vi "Phase_Shift_Keying.vi"() -> ()   [LabVIEW 2019]
panel:
  out "Modulated Signal":dbl[](graph)=[0.0, 0.40673664307580015, 0.7431448254773941, 0.9510565162951535, 0.9945218953682734, 0.8660254037844386, 0.5877852522924732, 0.20791169081775887, -0.20791169081775907, -0.5877852522924734, -0.8660254037844388, -0.9945218953682734, -0.9510565162951536, -0.7431448254773946, -0.4067366430757993, -2.4492935982947064e-16, 0.4067366430757997, 0.7431448254773948, 0.9510565162951538, 0.9945218953682733, 0.8660254037844383, 0.5877852522924734, 0.20791169081775912, -0.2079116908177584, -0.5877852522924728, -0.8660254037844387, -0.9945218953682732, -0.9510565162951538, -0.743144825477393, -0.40673664307579954, -4.898587196589413e-16, 0.40673664307580026, 0.7431448254773935, 0.9510565162951534, 0.9945218953682732, 0.8660254037844384, 0.5877852522924721, 0.20791169081775934, -0.2079116908177599, -0.5877852522924726, -0.8660254037844395, -0.9945218953682734, -0.9510565162951538, -0.7431448254773931, -0.40673664307579976, -7.347880794884119e-16, 0.40673664307579843, 0.7431448254773945, 0.9510565162951533, 0.9945218953682735, 0.8660254037844385, 0.5877852522924709, 0.2079116908177613, -0.20791169081775965, -0.5877852522924725, -0.8660254037844394, -0.9945218953682737, -0.9510565162951539, -0.7431448254773934, -0.4067366430758, -9.797174393178826e-16, 0.4067366430757982, 0.7431448254773944, 0.9510565162951543, 0.9945218953682736, 0.8660254037844386, 0.587785252292474, 0.2079116908177581, -0.2079116908177629, -0.5877852522924722, -0.8660254037844393, -0.9945218953682733, -0.9510565162951529, -0.7431448254773958, -0.4067366430758002, 2.328066879653148e-15, -0.40673664307580126, -0.7431448254773966, -0.9510565162951532, -0.9945218953682732, -0.8660254037844369, -0.5877852522924742, -0.20791169081775834, 0.2079116908177557, 0.587785252292472, 0.8660254037844392, 0.9945218953682737, 0.951056516295154, 0.7431448254773936, 0.4067366430757972, 1.4695761589768238e-15, -0.40673664307580104, -0.7431448254773916, -0.9510565162951531, -0.9945218953682733, -0.866025403784437, -0.5877852522924744, -0.20791169081775857, 0.20791169081775546, 0.5877852522924776, 0.866025403784439, 0.994521895368273, 0.9510565162951519, 0.7431448254773938, 0.4067366430758039, -5.3909218387947074e-15, -0.4067366430758008, -0.7431448254773915, -0.951056516295153, -0.9945218953682733, -0.8660254037844372, -0.5877852522924746, -0.20791169081775185, 0.20791169081776217, 0.5877852522924716, 0.8660254037844354, 0.9945218953682736, 0.9510565162951542, 0.7431448254773939, 0.40673664307579765, 1.959434878635765e-15, -0.40673664307580054, -0.7431448254773912, -0.9510565162951552, -0.9945218953682733, -0.8660254037844408, -0.587785252292469, -0.20791169081775904, 0.20791169081775498, 0.5877852522924714, 0.8660254037844388, 0.9945218953682736, 0.9510565162951542, 0.7431448254773941, 0.4067366430757979, 2.204364238465236e-15, -0.4067366430758068, -0.7431448254773959, -0.9510565162951529, -0.9945218953682733, -0.8660254037844374, -0.587785252292475, -0.2079116908177593, 0.20791169081776167, 0.587785252292477, 0.8660254037844386, 0.9945218953682728, 0.9510565162951521, 0.7431448254773942, 0.4067366430758046, -4.656133759306296e-15, 0.4067366430758001, 0.7431448254773958, 0.9510565162951506, 0.9945218953682726, 0.866025403784441, 0.5877852522924751, 0.20791169081775954, -0.20791169081776145, -0.5877852522924768, -0.866025403784442, -0.9945218953682743, -0.9510565162951544, -0.7431448254773945, -0.4067366430757983, 4.411204399476825e-15, 0.4067366430757934, 0.7431448254774004, 0.9510565162951528, 0.9945218953682734, 0.8660254037844377, 0.5877852522924696, 0.20791169081775282, -0.20791169081775426, -0.5877852522924708, -0.8660254037844384, -0.9945218953682735, -0.9510565162951566, -0.7431448254773898, -0.40673664307580504, -2.9391523179536475e-15, 0.40673664307579965, 0.7431448254773955, 0.9510565162951549, 0.9945218953682742, 0.8660254037844343, 0.5877852522924756, 0.20791169081776, -0.20791169081776098, -0.5877852522924764, -0.8660254037844418, -0.9945218953682727, -0.9510565162951545, -0.7431448254773853, -0.40673664307579876, 3.921345679817883e-15, 0.40673664307579294, 0.7431448254773905, 0.951056516295157, 0.9945218953682734, 0.8660254037844379, 0.58778525229247, 0.2079116908177672, -0.2079116908177538, -0.5877852522924819, -0.8660254037844382, -0.9945218953682735, -0.9510565162951524, -0.7431448254773997, -0.4067366430757925, 1.0781843677589415e-14, 0.4067366430757992, 0.7431448254773951, 0.9510565162951503, 0.9945218953682742, 0.8660254037844345, 0.587785252292476, 0.20791169081776048, -0.20791169081776048, -0.5877852522924645, -0.8660254037844416, -0.9945218953682742, -0.9510565162951546, -0.743144825477395, -0.4067366430757862, 3.4314869601589423e-15, -0.4067366430758055, -0.7431448254773901, -0.9510565162951524, -0.9945218953682735, -0.8660254037844453, -0.5877852522924705, -0.20791169081775376, 0.2079116908177533, 0.58778525229247, 0.866025403784445, 0.9945218953682734, 0.9510565162951525, 0.7431448254773905, 0.4067366430758059, 3.91886975727153e-15, -0.40673664307581175, -0.7431448254773948, -0.9510565162951545, -0.9945218953682743, -0.8660254037844418, -0.5877852522924649, -0.20791169081776095, 0.20791169081776, 0.5877852522924756, 0.8660254037844343, 0.9945218953682742, 0.9510565162951504, 0.7431448254773955, 0.40673664307579965, -2.941628240500001e-15, -0.40673664307579205, -0.7431448254773994, -0.9510565162951523, -0.9945218953682735, -0.8660254037844384, -0.5877852522924824, -0.20791169081775426, 0.20791169081776673, 0.5877852522924696, 0.8660254037844377, 0.9945218953682734, 0.9510565162951571, 0.7431448254773908, 0.4067366430757934, 4.408728476930472e-15, -0.4067366430757983, -0.743144825477404, -0.9510565162951544, -0.9945218953682728, -0.866025403784442, -0.5877852522924768, -0.20791169081774755, 0.20791169081775954, 0.5877852522924751, 0.866025403784441, 0.9945218953682726, 0.951056516295155, 0.7431448254773863, 0.4067366430758001, -2.45176952084106e-15, -0.4067366430758046, -0.7431448254773895, -0.9510565162951565, -0.9945218953682721, -0.8660254037844386, -0.5877852522924712, -0.20791169081776864, 0.20791169081775235, 0.5877852522924807, 0.8660254037844374, 0.9945218953682733, 0.9510565162951529, 0.7431448254774007, 0.4067366430757938]
  out "Carrier Signal":dbl[](graph)=[0.0, 0.40673664307580015, 0.7431448254773941, 0.9510565162951535, 0.9945218953682734, 0.8660254037844386, 0.5877852522924732, 0.20791169081775887, -0.20791169081775907, -0.5877852522924734, -0.8660254037844388, -0.9945218953682734, -0.9510565162951536, -0.7431448254773946, -0.4067366430757993, -2.4492935982947064e-16, 0.4067366430757997, 0.7431448254773948, 0.9510565162951538, 0.9945218953682733, 0.8660254037844383, 0.5877852522924734, 0.20791169081775912, -0.2079116908177584, -0.5877852522924728, -0.8660254037844387, -0.9945218953682732, -0.9510565162951538, -0.743144825477393, -0.40673664307579954, -4.898587196589413e-16, 0.40673664307580026, 0.7431448254773935, 0.9510565162951534, 0.9945218953682732, 0.8660254037844384, 0.5877852522924721, 0.20791169081775934, -0.2079116908177599, -0.5877852522924726, -0.8660254037844395, -0.9945218953682734, -0.9510565162951538, -0.7431448254773931, -0.40673664307579976, -7.347880794884119e-16, 0.40673664307579843, 0.7431448254773945, 0.9510565162951533, 0.9945218953682735, 0.8660254037844385, 0.5877852522924709, 0.2079116908177613, -0.20791169081775965, -0.5877852522924725, -0.8660254037844394, -0.9945218953682737, -0.9510565162951539, -0.7431448254773934, -0.4067366430758, -9.797174393178826e-16, 0.4067366430757982, 0.7431448254773944, 0.9510565162951543, 0.9945218953682736, 0.8660254037844386, 0.587785252292474, 0.2079116908177581, -0.2079116908177629, -0.5877852522924722, -0.8660254037844393, -0.9945218953682733, -0.9510565162951529, -0.7431448254773958, -0.4067366430758002, 2.328066879653148e-15, 0.40673664307580126, 0.7431448254773966, 0.9510565162951532, 0.9945218953682732, 0.8660254037844369, 0.5877852522924742, 0.20791169081775834, -0.2079116908177557, -0.587785252292472, -0.8660254037844392, -0.9945218953682737, -0.951056516295154, -0.7431448254773936, -0.4067366430757972, -1.4695761589768238e-15, 0.40673664307580104, 0.7431448254773916, 0.9510565162951531, 0.9945218953682733, 0.866025403784437, 0.5877852522924744, 0.20791169081775857, -0.20791169081775546, -0.5877852522924776, -0.866025403784439, -0.994521895368273, -0.9510565162951519, -0.7431448254773938, -0.4067366430758039, 5.3909218387947074e-15, 0.4067366430758008, 0.7431448254773915, 0.951056516295153, 0.9945218953682733, 0.8660254037844372, 0.5877852522924746, 0.20791169081775185, -0.20791169081776217, -0.5877852522924716, -0.8660254037844354, -0.9945218953682736, -0.9510565162951542, -0.7431448254773939, -0.40673664307579765, -1.959434878635765e-15, 0.40673664307580054, 0.7431448254773912, 0.9510565162951552, 0.9945218953682733, 0.8660254037844408, 0.587785252292469, 0.20791169081775904, -0.20791169081775498, -0.5877852522924714, -0.8660254037844388, -0.9945218953682736, -0.9510565162951542, -0.7431448254773941, -0.4067366430757979, -2.204364238465236e-15, 0.4067366430758068, 0.7431448254773959, 0.9510565162951529, 0.9945218953682733, 0.8660254037844374, 0.587785252292475, 0.2079116908177593, -0.20791169081776167, -0.587785252292477, -0.8660254037844386, -0.9945218953682728, -0.9510565162951521, -0.7431448254773942, -0.4067366430758046, 4.656133759306296e-15, 0.4067366430758001, 0.7431448254773958, 0.9510565162951506, 0.9945218953682726, 0.866025403784441, 0.5877852522924751, 0.20791169081775954, -0.20791169081776145, -0.5877852522924768, -0.866025403784442, -0.9945218953682743, -0.9510565162951544, -0.7431448254773945, -0.4067366430757983, 4.411204399476825e-15, 0.4067366430757934, 0.7431448254774004, 0.9510565162951528, 0.9945218953682734, 0.8660254037844377, 0.5877852522924696, 0.20791169081775282, -0.20791169081775426, -0.5877852522924708, -0.8660254037844384, -0.9945218953682735, -0.9510565162951566, -0.7431448254773898, -0.40673664307580504, -2.9391523179536475e-15, 0.40673664307579965, 0.7431448254773955, 0.9510565162951549, 0.9945218953682742, 0.8660254037844343, 0.5877852522924756, 0.20791169081776, -0.20791169081776098, -0.5877852522924764, -0.8660254037844418, -0.9945218953682727, -0.9510565162951545, -0.7431448254773853, -0.40673664307579876, 3.921345679817883e-15, 0.40673664307579294, 0.7431448254773905, 0.951056516295157, 0.9945218953682734, 0.8660254037844379, 0.58778525229247, 0.2079116908177672, -0.2079116908177538, -0.5877852522924819, -0.8660254037844382, -0.9945218953682735, -0.9510565162951524, -0.7431448254773997, -0.4067366430757925, 1.0781843677589415e-14, 0.4067366430757992, 0.7431448254773951, 0.9510565162951503, 0.9945218953682742, 0.8660254037844345, 0.587785252292476, 0.20791169081776048, -0.20791169081776048, -0.5877852522924645, -0.8660254037844416, -0.9945218953682742, -0.9510565162951546, -0.743144825477395, -0.4067366430757862, 3.4314869601589423e-15, 0.4067366430758055, 0.7431448254773901, 0.9510565162951524, 0.9945218953682735, 0.8660254037844453, 0.5877852522924705, 0.20791169081775376, -0.2079116908177533, -0.58778525229247, -0.866025403784445, -0.9945218953682734, -0.9510565162951525, -0.7431448254773905, -0.4067366430758059, -3.91886975727153e-15, 0.40673664307581175, 0.7431448254773948, 0.9510565162951545, 0.9945218953682743, 0.8660254037844418, 0.5877852522924649, 0.20791169081776095, -0.20791169081776, -0.5877852522924756, -0.8660254037844343, -0.9945218953682742, -0.9510565162951504, -0.7431448254773955, -0.40673664307579965, 2.941628240500001e-15, 0.40673664307579205, 0.7431448254773994, 0.9510565162951523, 0.9945218953682735, 0.8660254037844384, 0.5877852522924824, 0.20791169081775426, -0.20791169081776673, -0.5877852522924696, -0.8660254037844377, -0.9945218953682734, -0.9510565162951571, -0.7431448254773908, -0.4067366430757934, -4.408728476930472e-15, 0.4067366430757983, 0.743144825477404, 0.9510565162951544, 0.9945218953682728, 0.866025403784442, 0.5877852522924768, 0.20791169081774755, -0.20791169081775954, -0.5877852522924751, -0.866025403784441, -0.9945218953682726, -0.951056516295155, -0.7431448254773863, -0.4067366430758001, 2.45176952084106e-15, 0.4067366430758046, 0.7431448254773895, 0.9510565162951565, 0.9945218953682721, 0.8660254037844386, 0.5877852522924712, 0.20791169081776864, -0.20791169081775235, -0.5877852522924807, -0.8660254037844374, -0.9945218953682733, -0.9510565162951529, -0.7431448254774007, -0.4067366430757938]
  out "Modulating Signal":dbl[](graph)=[0.0, 1.0, 1.0, 1.0, 1.0, 1.0, 1.0, 1.0, 1.0, 1.0, 1.0, 1.0, 1.0, 1.0, 1.0, 1.0, 1.0, 1.0, 1.0, 1.0, 1.0, 1.0, 1.0, 1.0, 1.0, 1.0, 1.0, 1.0, 1.0, 1.0, 1.0, 1.0, 1.0, 1.0, 1.0, 1.0, 1.0, 1.0, 1.0, 1.0, 1.0, 1.0, 1.0, 1.0, 1.0, 1.0, 1.0, 1.0, 1.0, 1.0, 1.0, 1.0, 1.0, 1.0, 1.0, 1.0, 1.0, 1.0, 1.0, 1.0, 1.0, 1.0, 1.0, 1.0, 1.0, 1.0, 1.0, 1.0, 1.0, 1.0, 1.0, 1.0, 1.0, 1.0, 1.0, 1.0, -1.0, -1.0, -1.0, -1.0, -1.0, -1.0, -1.0, -1.0, -1.0, -1.0, -1.0, -1.0, -1.0, -1.0, -1.0, -1.0, -1.0, -1.0, -1.0, -1.0, -1.0, -1.0, -1.0, -1.0, -1.0, -1.0, -1.0, -1.0, -1.0, -1.0, -1.0, -1.0, -1.0, -1.0, -1.0, -1.0, -1.0, -1.0, -1.0, -1.0, -1.0, -1.0, -1.0, -1.0, -1.0, -1.0, -1.0, -1.0, -1.0, -1.0, -1.0, -1.0, -1.0, -1.0, -1.0, -1.0, -1.0, -1.0, -1.0, -1.0, -1.0, -1.0, -1.0, -1.0, -1.0, -1.0, -1.0, -1.0, -1.0, -1.0, -1.0, -1.0, -1.0, -1.0, -1.0, 1.0, 1.0, 1.0, 1.0, 1.0, 1.0, 1.0, 1.0, 1.0, 1.0, 1.0, 1.0, 1.0, 1.0, 1.0, 1.0, 1.0, 1.0, 1.0, 1.0, 1.0, 1.0, 1.0, 1.0, 1.0, 1.0, 1.0, 1.0, 1.0, 1.0, 1.0, 1.0, 1.0, 1.0, 1.0, 1.0, 1.0, 1.0, 1.0, 1.0, 1.0, 1.0, 1.0, 1.0, 1.0, 1.0, 1.0, 1.0, 1.0, 1.0, 1.0, 1.0, 1.0, 1.0, 1.0, 1.0, 1.0, 1.0, 1.0, 1.0, 1.0, 1.0, 1.0, 1.0, 1.0, 1.0, 1.0, 1.0, 1.0, 1.0, 1.0, 1.0, 1.0, 1.0, 1.0, -1.0, -1.0, -1.0, -1.0, -1.0, -1.0, -1.0, -1.0, -1.0, -1.0, -1.0, -1.0, -1.0, -1.0, -1.0, -1.0, -1.0, -1.0, -1.0, -1.0, -1.0, -1.0, -1.0, -1.0, -1.0, -1.0, -1.0, -1.0, -1.0, -1.0, -1.0, -1.0, -1.0, -1.0, -1.0, -1.0, -1.0, -1.0, -1.0, -1.0, -1.0, -1.0, -1.0, -1.0, -1.0, -1.0, -1.0, -1.0, -1.0, -1.0, -1.0, -1.0, -1.0, -1.0, -1.0, -1.0, -1.0, -1.0, -1.0, -1.0, -1.0, -1.0, -1.0, -1.0, -1.0, -1.0, -1.0, -1.0, -1.0, -1.0, -1.0, -1.0, -1.0, -1.0]
  in  "fm":dbl=20.0
  out "No. of\nsamples":dbl=300.0
  in  "No. of\ncycles":dbl=2.0
  in  "fs":dbl=3000.0
  in  "fc":dbl=200.0
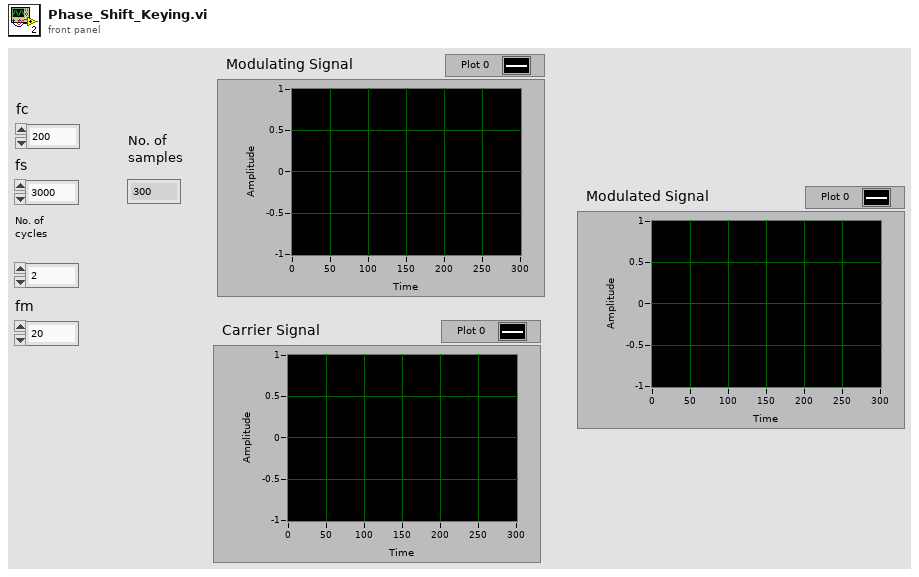
[diagram p1: front panel]
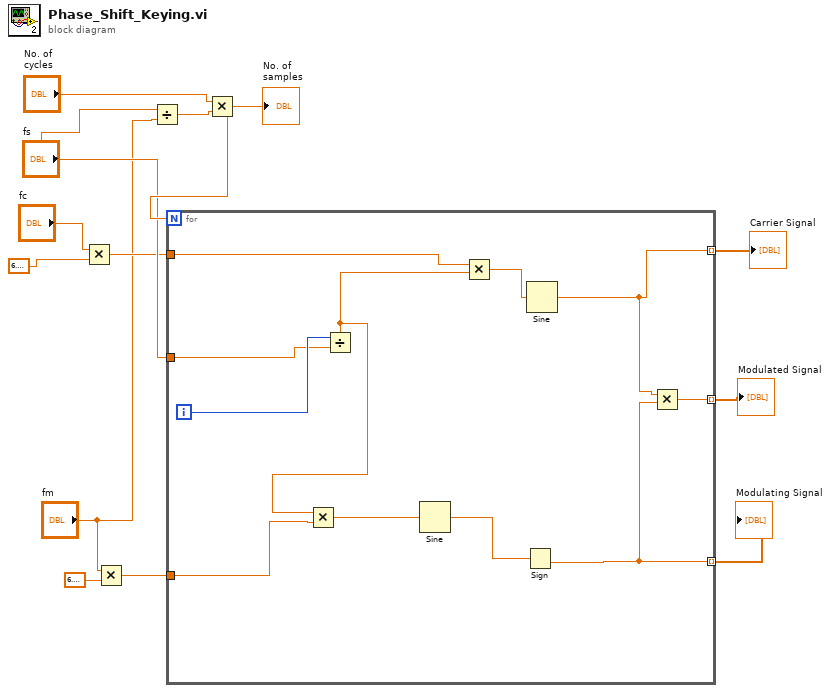
[diagram p0: block diagram]
diagram:
  n1 = Multiply(x="fc", y=6.283185307179586) -> (x*y=w6:dbl)
  n2 = Multiply(x="fm", y=6.283185307179586) -> (x*y=w7:dbl)
  n3 = Divide(x="fs", y="fm") -> (x/y=w13:dbl)
  n4 = Multiply(x="No. of\ncycles", y=w13) -> (x*y=w11:dbl)
  "No. of\nsamples" <- w11
  n5 = for {
    N: w11 -> [_]
    tunnel: "fs" -> [w23]
    tunnel: w7 -> [w22]
    tunnel: w6 -> [w19]
    tunnel: [w17] -> w3 mode=indexing
    tunnel: [w14] -> w2 mode=indexing
    tunnel: [w16] -> w1 mode=indexing
    i -> [w24]
    n6 = Divide(x=w24, y=w23) -> (x/y=w18:dbl)
    n7 = Multiply(x=w18, y=w22) -> (x*y=w21:dbl)
    n8 = Sine(x=w21) -> (sin(x)=w15:dbl)
    n9 = Multiply(x=w19, y=w18) -> (x*y=w20:dbl)
    n10 = Sign(1:w15) -> (0:w14:dbl)
    n11 = Sine(x=w20) -> (sin(x)=w17:dbl)
    n12 = Multiply(x=w17, y=w14) -> (x*y=w16:dbl)
  }
  "Modulating Signal" <- w2
  "Carrier Signal" <- w3
  "Modulated Signal" <- w1
